vi "Asylum_SetOutWave.vi"(6 "interpolation":i32, 7 "whichBank":i32, 8 "error in (no error)":errorcluster, 9 "Wave":cluster{"channelString":string, "wave":string}, 10 "eventString":string, 11 "Application":refnum<k7>) -> (0 "error out":errorcluster, 3 "Application":refnum<k7>)   [LabVIEW 2019]
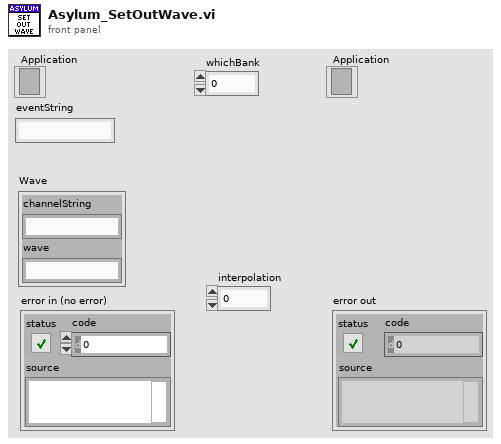
[diagram p1: front panel]
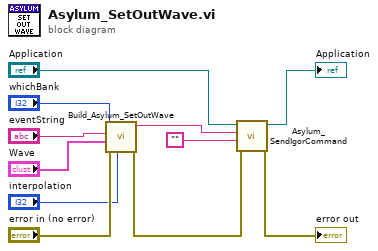
[diagram p0: block diagram]
diagram:
  n1 = call "Build_Asylum_SetOutWave.vi"("interpolation"="interpolation", "error in (no error)"="error in (no error)", "Wave"="Wave", "eventString"="eventString", "whichBank"="whichBank") -> ("error out"=w11:errorcluster, "Command"=w9:string)  [unwired: 5 in]
  n2 = call "Asylum_SendIgorCommand.vi"("error in (no error)"=w11, "Format"="", "command"=w9, "Application In"="Application") -> ("error out"=→"error out":errorcluster, "Application Out"=→"Application":refnum<k7>)  [unwired: 4 in, 2 out]
